vi "copyright.vi"() -> ()   [LabVIEW 2012, in "Design Server.lvlib"]
uses:
  Design Server.lvlib
  help.ctl
  <vilib>/Platform/browser.llb/Open URL in Default Browser (string).vi
panel:
  in  "Help Button":T1
  in  "OK Button":bool
  out "Info":string
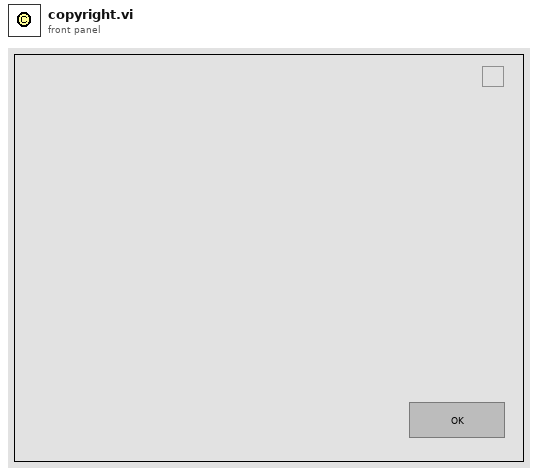
[diagram p1: front panel]
types:
  T1 = typedef "Design Server.lvlib/help.ctl" = bool
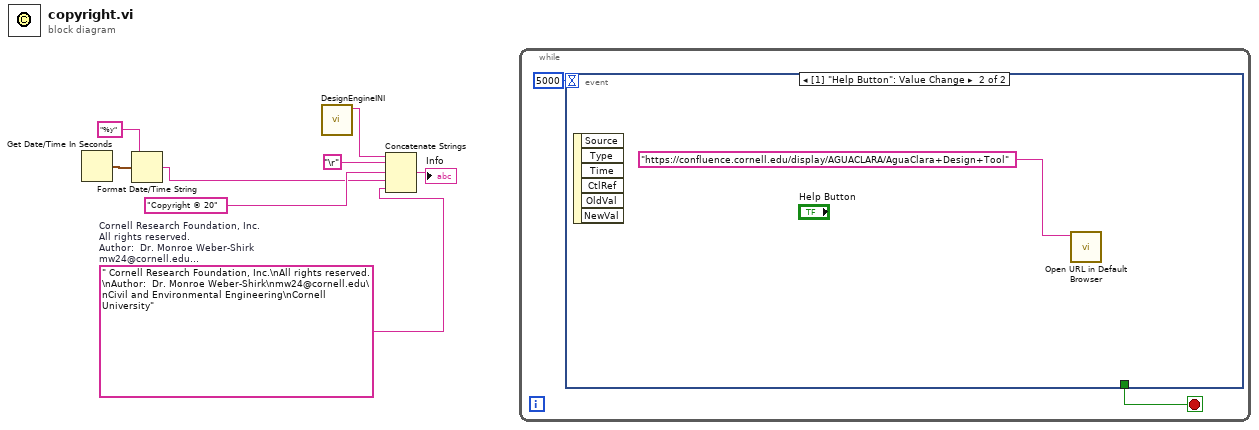
[diagram p0: block diagram]
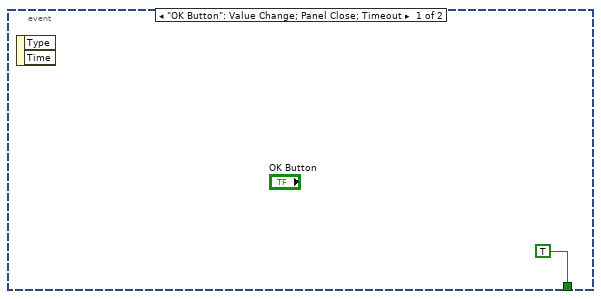
[diagram p2: hidden frame]
diagram:
  w8 = " Cornell Research Foundation, Inc.\nAll rights reserved.\nAuthor:  Dr. Monroe Weber-Shirk\nmw24@cornell.edu\nCivil and Environmental Engineering\nCornell University"  # Cornell Research Foundation, Inc. All rights reserved. Author:  Dr. Monroe Weber-Shirk mw24@cornell.edu Civil and Environmental Engineering Cornell University
  n1 = Get Date/Time In Seconds() -> (seconds since 1Jan1904=w4:timestamp)
  n2 = Format Date/Time String(time format string (%c)="%y", seconds (now)=w4) -> (date/time string=w1:string)  [unwired: 1 in]
  n3 = call "DesignEngineINI.vi"() -> ("Application Name"=w5:string)  [unwired: 6 in, 1 out]
  n4 = Concatenate Strings(w5, "\r", "Copyright © 20", w1, w8) -> (→"Info":string)
  n5 = while {
    stop <- w10 stop-if-true
    n6 = event shown="[1] \"Help Button\": Value Change" {
      selector: _ -> [_ _]
      dyn-events: _ -> [_ _]
      timeout: 5000 -> [_ _]
      tunnel: [TRUE _] -> w10
      event "OK Button": Value Change; Panel Close; Timeout {
        n7 = event-data() -> ()  [unwired: 1 in, 2 out]
      }
      event Value Change {
        n8 = event-data() -> ()  [unwired: 1 in, 6 out]
        n9 = call-poly <vilib>:"Open URL in Default Browser.vi"("URL"="https://confluence.cornell.edu/display/AGUACLARA/AguaClara+Design+Tool") -> ()  [unwired: 5 in, 2 out]
      }
    }
  }
